vi "AttributeArrayToString.vi"(8 "error in (no error)":errorcluster, 10 "Array":T1[](array[typedef])=[{"attributeType"="", "attributeValue"=""}], 11 "WriteAttribute in":refnum<class "XMLAttributeGenerator.lvclass">) -> (0 "error out":errorcluster, 2 "attributeString":string, 3 "WriteAttribute out":refnum<class "XMLAttributeGenerator.lvclass">)   [LabVIEW 2014, in "XML.lvlib" / "XMLAttributeGenerator.lvclass"]
doc: "This method calls the format attribute for an array of attributes"
uses:
  <userlib>/Common/XML/XMLAttributeGenerator/XMLAttributeGenerator.lvclass
  <userlib>/Common/XML/Typedefs/AttributeElements.ctl
  <vilib>/dlg_ctls.llb/Space Constant.vi
  <userlib>/Common/XML/XML.lvlib
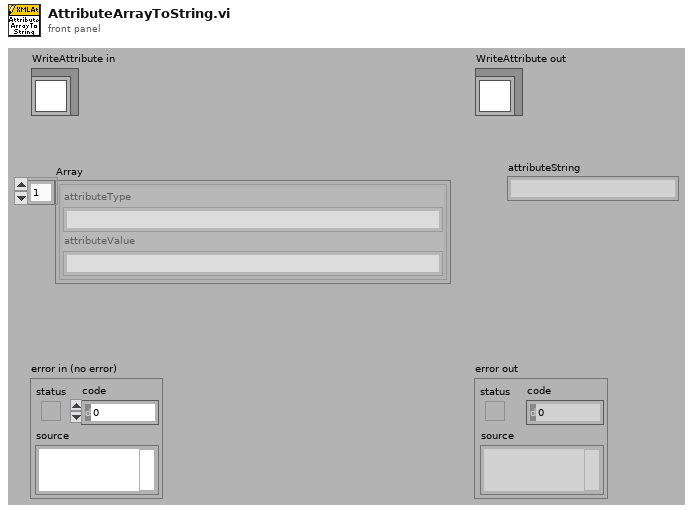
[diagram p1: front panel]
types:
  T1 = typedef "XML.lvlib/AttributeElements.ctl" = cluster{"attributeType":string, "attributeValue":string}
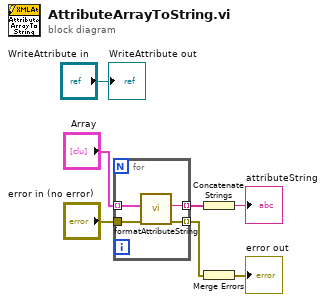
[diagram p0: block diagram]
diagram:
  n1 = for {
    tunnel: "Array" -> [w11] mode=indexing
    tunnel: [w10] -> w5 mode=indexing
    tunnel: "error in (no error)" -> [w9]
    tunnel: [w8] -> w2 mode=indexing
    n2 = call <userlib>:"formatAttributeString.vi"("error in (no error)"=w9, "attributeElement"=w11) -> ("error out"=w8:errorcluster, "String"=w10:string)  [unwired: 7 in, 1 out]
  }
  n3 = Concatenate Strings(w5) -> (→"attributeString":string)
  n4 = Merge Errors(w2) -> (→"error out":errorcluster)
  "WriteAttribute out" <- "WriteAttribute in"
